vi "Data.vi"(11 "Set Error Msg in":refnum<class "Set Error Msg.lvclass">) -> (2 "Error":errorcluster)   [LabVIEW 2021, in "Set Error.lvlib" / "Set Error Msg.lvclass"]
uses:
  Set Error Msg.lvclass
  Set Error Msg.lvclass/Set Error Msg.ctl
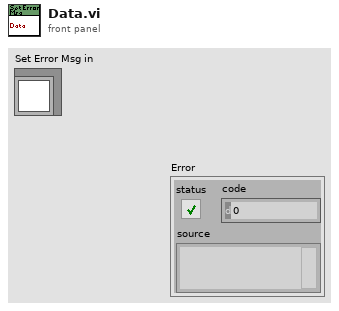
[diagram p1: front panel]
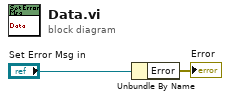
[diagram p0: block diagram]
diagram:
  n1 = Unbundle By Name("Set Error Msg in") -> ("Error"=→"Error":errorcluster)
